vi "Read Errors.vi"(0 "FPGA API in":refnum<class "FPGA API Mock.lvclass">, 11 "error in (no error)":errorcluster) -> (4 "FPGA API out":refnum<class "FPGA API Mock.lvclass">, 8 "Errors":errorcluster[](array[cluster]), 15 "error out":errorcluster)   [LabVIEW 2019, in "FPGA API Mock.lvclass"]
uses:
  FPGA API Mock.lvclass
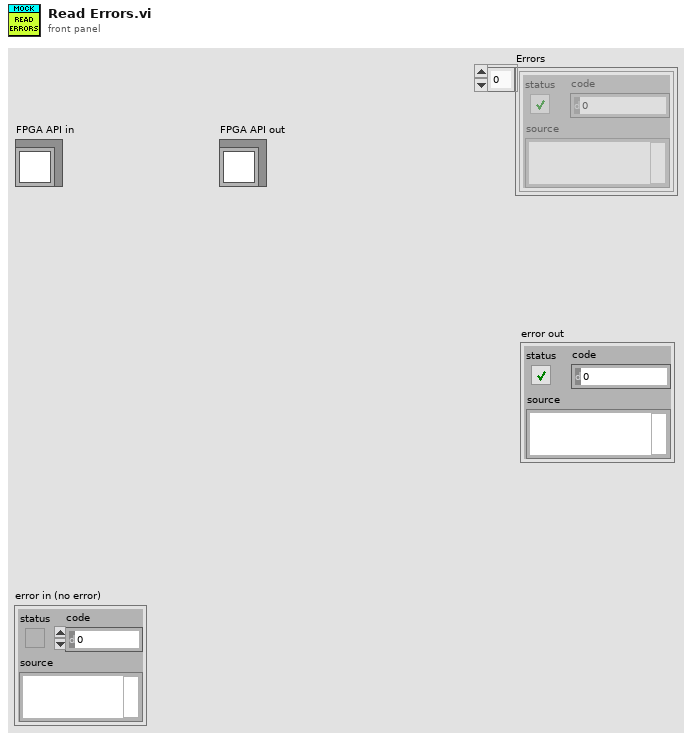
[diagram p1: front panel]
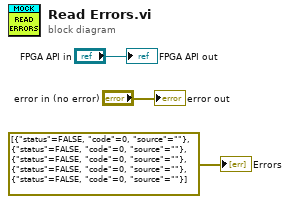
[diagram p0: block diagram]
diagram:
  "FPGA API out" <- "FPGA API in"
  "Errors" <- errorcluster[] [{"status"=FALSE, "code"=0, "source"=""}, {"status"=FALSE, "code"=0, "source"=""}, {"status"=FALSE, "code"=0, "source"=""}, {"status"=FALSE, "code"=0, "source"=""}, {"status"=FALSE, "code"=0, "source"=""}] ("Errors")
  "error out" <- "error in (no error)"
